vi "PH_DataViewer.write Data to Harddisk.vi"(1 "error in":errorcluster, 2 "String":string) -> (0 "error out":errorcluster)   [LabVIEW 2014, in "PH_DataViewer.lvlib"]
doc: "This VI writes string data to the harddrive. Defaut path starts with \"O:\\\"."
uses:
  PH_DataViewer.lvlib
  PH_Common/Names/PH_Names.File Types.ctl
  PH_Common/PH_Common.lvlib
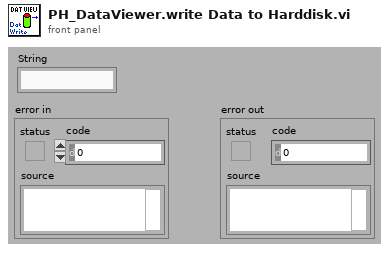
[diagram p1: front panel]
types:
  T1 = typedef "PH_Common.lvlib/PH_Names.File Types.ctl" = string
  T2 = enum16{"open", "replace", "create", "open or create", "replace or create", "replace or create with confirmation"}
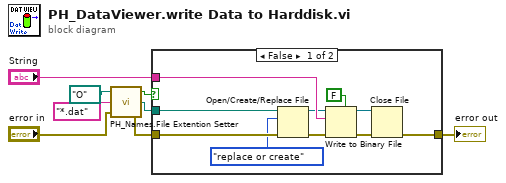
[diagram p0: block diagram]
diagram:
  n1 = call "PH_Names.File Extention Setter.vi"("error in (no error)"="error in", "File Type"=T1 "*.dat" ("file name extention"), "start path (O:\\)"=path "O:/" ("start path (O:\\)")) -> ("error out"=w1:errorcluster, "path with extension"=w4:path, "cancelled?"=w8:bool)
  n2 = case shown="False" w8 {
    tunnel: "String" -> [w18 _]
    tunnel: w4 -> [w13 _]
    tunnel: [w11 w19] -> w5
    tunnel: w1 -> [w10 w19]
    frame False {
      n3 = Open/Create/Replace File(file path (use dialog)=w13, error in=w10, operation (0:open)=T2."replace or create") -> (refnum out=w14:refnum<file>, error out=w16:errorcluster)  [unwired: 3 in, 1 out]
      n4 = Write to Binary File(file (use dialog)=w14, data=w18, error in=w16, 5:FALSE ("prepend array or string size? (T)")) -> (refnum out=w17:refnum<file>, error out=w15:errorcluster)  [unwired: 2 in, 1 out]
      n5 = Close File(refnum=w17, error in=w15) -> (error out=w11:errorcluster)  [unwired: 1 out]
    }
    frame True {
    }
  }
  "error out" <- w5
